vi "Random Change Flag.vi"() -> (0 "Random Change Flag":u64=4603270806574966694 format="%08x")   [LabVIEW 2017, in "Communicable State Machine.lvlib"]
doc: "### Random Change Flag.vi\n\nGenerate a random value to mark state changes. In CSM, this flag is used in some places to determine whether the cache needs to be updated for efficiency.\n\n-- <b>Indicators</b> --\n- <b>Random Change Flag</b>: Generated random value"
uses:
  Communicable State Machine.lvlib
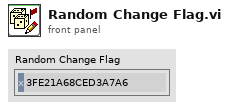
[diagram p1: front panel]
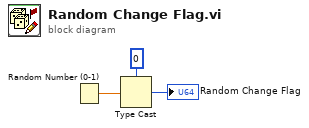
[diagram p0: block diagram]
diagram:
  n1 = Random Number (0-1)() -> (number: 0 to 1=w3:dbl)
  n2 = Type Cast(type=u64 0 ("global-CSMQ FGV Change Flag"), x=w3) -> (*(type *) &x=→"Random Change Flag":u64)
